vi "RRR_Trajectory_Generation_2025.vi"() -> ()   [LabVIEW 2020]
panel:
  in  "Show Path?":bool
  in  "Claw Value (End)":dbl=1.0
  in  "Claw Value (Start)":dbl
  in  "TCP (End)":dbl=90.0
  in  "TCP (Start)":dbl
  in  "Psi_deg (End)":dbl=90.0
  in  "Psi_deg (Start)":dbl
  in  "Y (Start Position)":dbl=20.0
  in  "X (Start Position)":dbl=60.0
  in  "Steps":dbl=100.0
  in  "Y (End Position)":dbl=-20.0
  in  "X (End Position)":dbl=60.0
  in  "Scale Factor":dbl(slide)=0.7 scale=0.5..1.0
  out "RRR - Trajectory Generation":picture
  in  "Add details":bool=TRUE
  in  "Light Direction":dbl(knob)=5.611498737356196 scale format="%#.1f"
  in  "Colors":T1={"Joint 1"=16750848, "Arm 1"=16764006, "Joint 2"=26316, "Arm B"=6723993, "Joint 4"=16724787, "Claw"=16776960, "Joint 3"=26316, "Arm C"=6723993}
  in  "Elbow Up?":bool
  out "Theta_3":dbl=-90.89511635103433
  out "Theta_2":dbl=126.83471722543209
  out "Theta_1":dbl=-35.20973591447286
  out "Y_Target":dbl=1.4141414141414153
  out "Y_Wrist":dbl=1.159377371477102
  out "Y_Elbow":dbl=-28.82855800916939
  out "X_Target":dbl=60.0
  out "X_Wrist":dbl=40.00162268376343
  out "X_Elbow":dbl=40.85234684950126
  in  "L3":dbl=20.0
  out "RRR - Trajectory Generation":cluster{dbl[], dbl[]}[](graph)=[{[0.0, 40.85234684950126, 40.00162268376343, 60.0], [0.0, -28.82855800916939, 1.159377371477102, 1.4141414141414153]}, {[], []}]
  in  "L2":dbl=30.0
  in  "L1":dbl=50.0
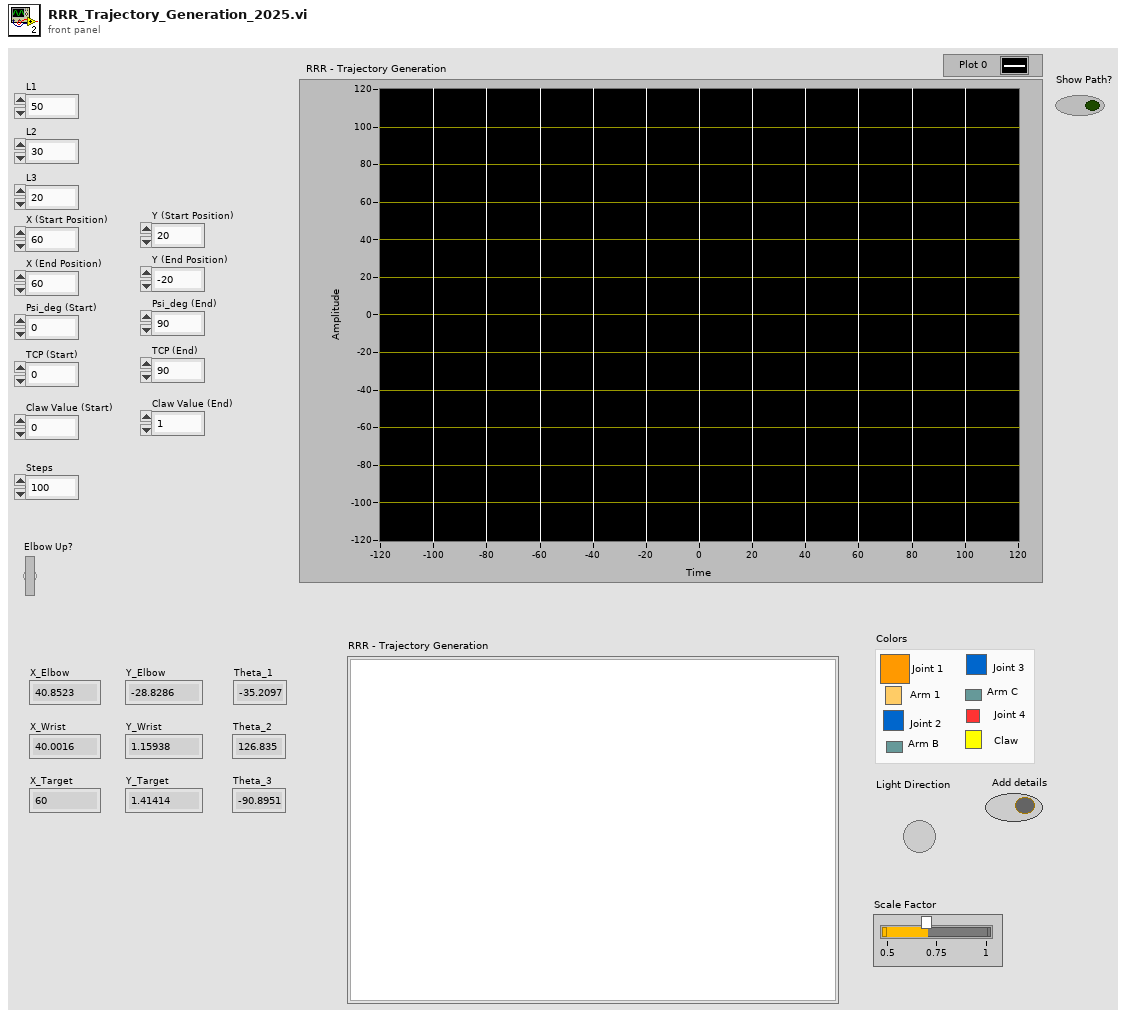
[diagram p1: front panel]
types:
  T1 = cluster{"Joint 1":u32, "Arm 1":u32, "Joint 2":u32, "Arm B":u32, "Joint 4":u32, "Claw":u32, "Joint 3":u32, "Arm C":u32}
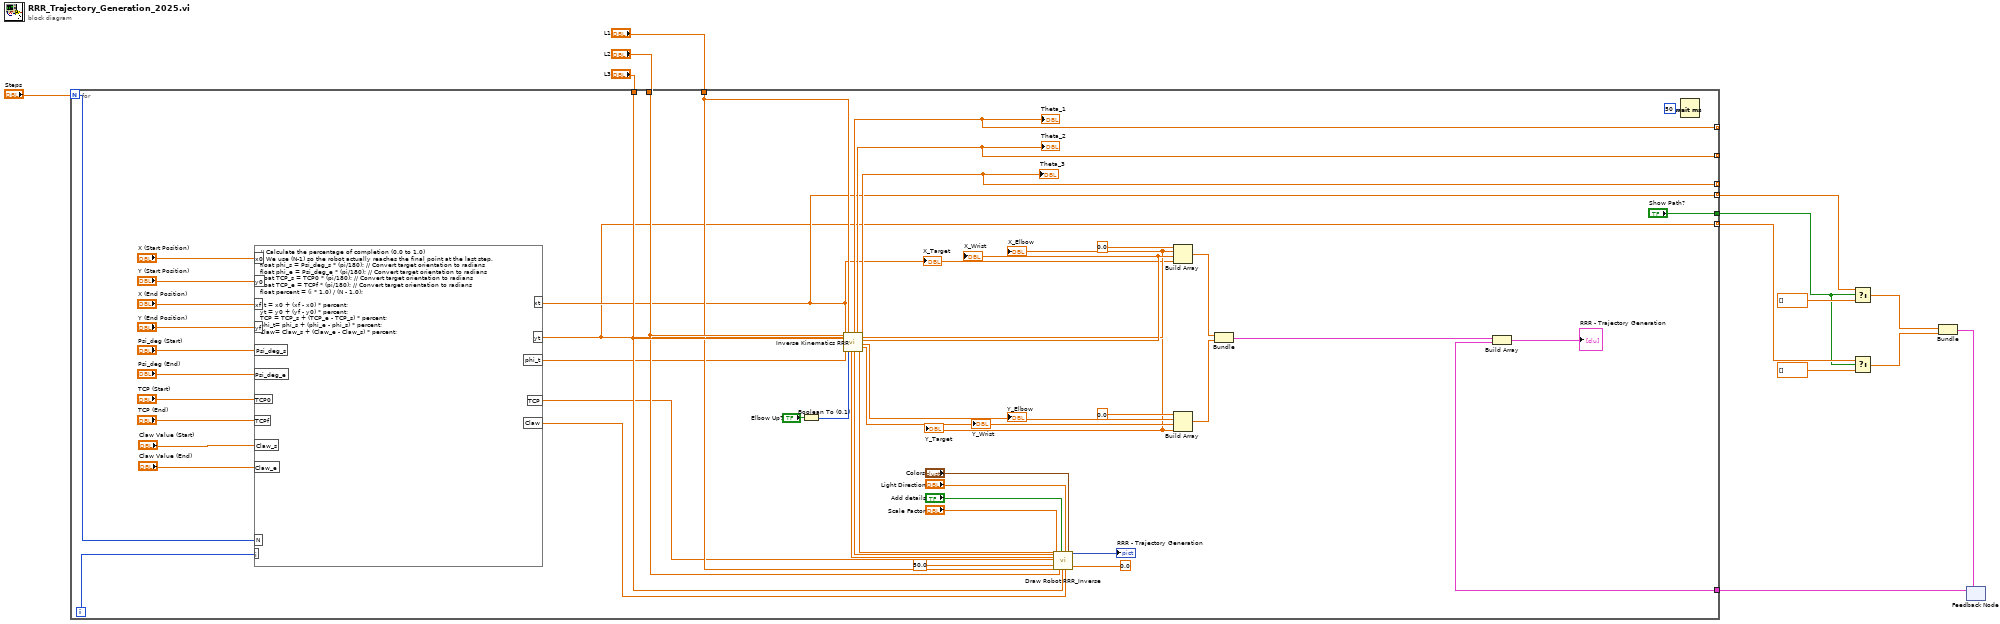
[diagram p0: block diagram]
diagram:
  n1 = feedback #1() -> (w4:cluster{"f":dbl[], "f":dbl[]})  [unwired: 1 in]
  n2 = for {
    N: "Steps" -> [w56]
    tunnel: "L3" -> [w36]
    tunnel: "L2" -> [w35]
    tunnel: "L1" -> [w34]
    tunnel: [w33] -> _ mode=indexing
    tunnel: [w32] -> _ mode=indexing
    tunnel: [w31] -> _ mode=indexing
    tunnel: [w19] -> w6 mode=indexing
    tunnel: [w18] -> w5 mode=indexing
    tunnel: w4 -> [w16]
    tunnel: ["Show Path?"] -> w1
    i -> [w57]
    n3 = formula code="// Calculate the percentage of completion (0.0 to 1.0)\n// We use (N-1) so the robot actually reaches the final point at the last step.\nfloat phi_s = Psi_deg_s * (pi/180); // Convert target orientation to radians\nfloat phi_e = Psi_deg_e * (pi/180); // Convert target orientation to radians\nfloat TCP_s = TCP0 * (pi/180); // Convert target orientation to radians\nfloat TCP_e = TCPf * (pi/180); // Convert target orientation to radians\nfloat percent = (i * 1.0) / (N - 1.0);\n\nxt = x0 + (xf - x0) * percent;\nyt = y0 + (yf - y0) * percent;\nTCP = TCP_s + (TCP_e - TCP_s) * percent;\nphi_t= phi_s + (phi_e - phi_s) * percent;\nClaw= Claw_s + (Claw_e - Claw_s) * percent;"("x0"="X (Start Position)", "y0"="Y (Start Position)", "xf"="X (End Position)", "yf"="Y (End Position)", "i"=w57, "N"=w56, "Psi_deg_s"="Psi_deg (Start)", "Psi_deg_e"="Psi_deg (End)", "TCP0"="TCP (Start)", "TCPf"="TCP (End)", "Claw_s"="Claw Value (Start)", "Claw_e"="Claw Value (End)") -> ("xt"=w19:dbl, "yt"=w18:dbl, "phi_t"=w28:dbl, "TCP"=w24:dbl, "Claw"=w23:dbl)
    "X_Target" <- w19
    "Y_Target" <- w18
    n4 = Boolean To (0,1)(Boolean="Elbow Up?") -> (0, 1=w48:i16)
    n5 = call "Inverse Kinematics RRR.vi"("L2"=w35, "L3"=w36, "X (Target Position)"=w19, "Y (Target Position)"=w18, "Psi (Target Orientation)"=w28, "L1"=w34, "Numeric 4"=w48) -> ("Numeric"=w55:dbl, "th1_deg"=w33:dbl, "Numeric 3"=w53:dbl, "th2_deg"=w32:dbl, "Numeric 2"=w54:dbl, "th3_deg"=w31:dbl, "x_elbow"=w41:dbl, "x_wrist"=w44:dbl, "y_elbow"=w46:dbl, "y_wrist"=w45:dbl)  [unwired: 3 in]
    "X_Elbow" <- w41
    "X_Wrist" <- w44
    "Y_Elbow" <- w46
    "Y_Wrist" <- w45
    "Theta_1" <- w33
    "Theta_2" <- w32
    "Theta_3" <- w31
    n6 = call "Draw Robot RRR_Inverse.vi"("Scale Factor"="Scale Factor", "Numeric 3"=w53, "TCP"=w24, "Numeric"=w55, "y 2"=50.0 ("y"), "L1"=w34, "Numeric 2"=w54, "L2"=w35, "Add details"="Add details", "L3"=w36, "Light Direction"="Light Direction", "Claw Value"=w23, "Colors"="Colors", "y"=0.0) -> ("Picture Out"=→"RRR - Trajectory Generation":picture)  [unwired: 5 in]
    n7 = Build Array(0.0 ("element"), w41, w44, w19) -> (w42:dbl[])
    n8 = Build Array(0.0 ("element"), w46, w45, w18) -> (w43:dbl[])
    n9 = Bundle(w42, w43) -> (w17:cluster{dbl[], dbl[]})  [unwired: 1 in]
    n10 = Build Array(w17, w16) -> (→"RRR - Trajectory Generation":cluster{"f":dbl[], "f":dbl[]}[])
    n11 = Wait (ms)(milliseconds to wait=u32 50) -> ()  [unwired: 1 out]
  }
  n12 = Select(t=w6, s=w1, f=dbl[] []) -> (s? t:f=w9:dbl[])
  n13 = Select(t=w5, s=w1, f=dbl[] []) -> (s? t:f=w8:dbl[])
  n14 = Bundle("f"=w9, "f"=w8) -> (w7:cluster{"f":dbl[], "f":dbl[]})  [unwired: 1 in]
  n15 = feedback-in #1(w7) -> ()
